vi "pthread_mutex_lock.vi"(8 "error in (no error)":errorcluster, 11 "mutex ptr in":u64) -> (0 "error out":errorcluster, 3 "mutex ptr out":u64)   [LabVIEW 2013, in "POSIX Threads.lvlib" / "POSIX Thread Object.lvclass"]
uses:
  POSIX Thread Object.lvclass
  Controls/pthread functions.ctl
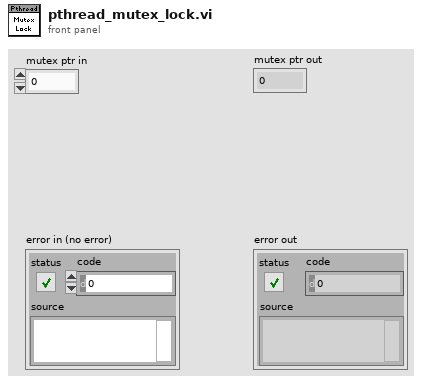
[diagram p1: front panel]
types:
  T1 = typedef "POSIX Threads.lvlib/POSIX Thread Object.lvclass/pthread functions.ctl" = enum16{"unspecified", "pthread_condattr_init", "pthread_condattr_destroy", "pthread_condattr_getclock", "pthread_condattr_setclock", "pthread_condattr_getpshared", "pthread_condattr_setpshared", "pthread_cond_init", "pthread_cond_destroy", "pthread_cond_broadcast", "pthread_cond_signal", "pthread_cond_timedwait", "pthread_cond_wait", "pthread_mutexattr_init", "pthread_mutexattr_destroy", "pthread_mutexattr_getprioceiling", "pthread_mutexattr_setprioceiling", "pthread_mutexattr_getprotocol", "pthread_mutexattr_setprotocol", "pthread_mutexattr_getpshared", "pthread_mutexattr_setpshared", "pthread_mutexattr_gettype", "pthread_mutexattr_settype", "pthread_mutex_init", "pthread_mutex_destroy", "pthread_mutex_getprioceiling", "pthread_mutex_setprioceiling", "pthread_mutex_lock", "pthread_mutex_timedlock", "pthread_mutex_trylock", "pthread_mutex_unlock", "sem_destroy", "sem_getvalue", "sem_init", "sem_post", "sem_timedwait", "sem_trywait", "sem_wait", "barrier_init", "barrier_destroy", "barrier_wait", "barrierattr_init", "barrierattr_destroy", "barrierattr_getpshared", "barrierattr_setpshared"}
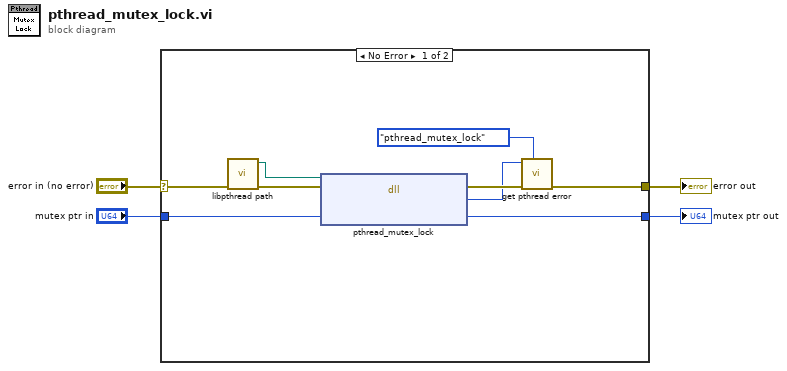
[diagram p0: block diagram]
diagram:
  n1 = case shown="No Error" "error in (no error)" {
    selector: "error in (no error)" -> [w13 w15]
    tunnel: "mutex ptr in" -> [w12 w14]
    tunnel: [w11 w15] -> w2
    tunnel: [w10 w14] -> w1
    frame No Error {
      n2 = call "libpthread path.vi"("error in (no error)"=w13) -> ("error out"=w8:errorcluster, "path to libpthread"=w9:path)  [unwired: 9 in]
      n3 = dll-call lib="?" fn="pthread_mutex_lock"(path in=w9, error in=w8, "mutex"=w12) -> (error out=w7:errorcluster, "errno"=w5:i32, "mutex"=w10:u64)  [unwired: 1 in, 1 out]
      n4 = call "get pthread error.vi"("function"=pthread_functions."pthread_mutex_lock", "error in (no error)"=w7, "errno"=w5) -> ("error out"=w11:errorcluster)  [unwired: 8 in]
    }
    frame Error {
    }
  }
  "error out" <- w2
  "mutex ptr out" <- w1
